vi "Control Spring.vi"   [LabVIEW 2020]
uses:
  Framework/Robot Global Data.vi
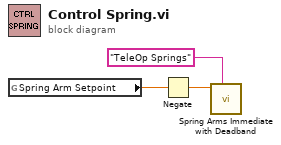
[diagram p0: block diagram]
diagram:
  n1 = global read "Robot Global Data.vi" "Spring Arm Setpoint"() -> (w1:dbl)
  n2 = Negate(x=w1) -> (-x=w2:dbl)
  n3 = call "Spring Arms Immediate with Deadband.vi"("Description"="TeleOp Springs", "Setpoint"=w2) -> ()  [unwired: 9 in, 1 out]
